vi "fpga_2CH Output Valid.vi"(2 "output valid":bool, 3 "1CH?":bool) -> (0 "output valid":bool)   [LabVIEW 2011, in "NI_EP_Resample_FPGA.lvlib"]
uses:
  <vilib>/addons/Electrical Power/PQ/Resampling/NI_EP_Resample_FPGA.lvlib
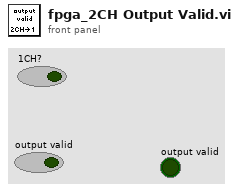
[diagram p1: front panel]
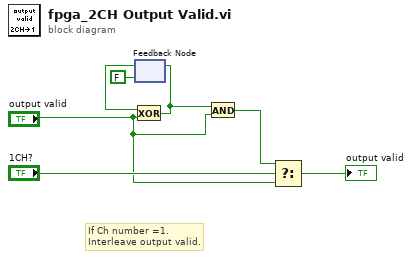
[diagram p0: block diagram]
diagram:
  # "If Ch number =1.\nInterleave output valid."
  n1 = feedback #1(FALSE ("s")) -> (w5:bool)
  n2 = Exclusive Or(1:"output valid", 2:w5) -> (0:w4:bool)
  n3 = feedback-in #1(w4) -> ()
  n4 = And(x=w4, y="output valid") -> (x .and. y?=w3:bool)
  n5 = Select(t=w3, s="1CH?", f="output valid") -> (s? t:f=→"output valid":bool)
